vi "openOrigin.vi"   [LabVIEW 2015]
uses:
  <vilib>/registry/registry.llb/Registry RtKey.ctl
  <vilib>/registry/registry.llb/Registry SAM.ctl
  <vilib>/registry/registry.llb/Registry View.ctl
  <vilib>/registry/registry.llb/Read Registry Value Simple STR.vi
types:
  T1 = typedef "Registry View.ctl" = u16
  T2 = typedef "Registry SAM.ctl" = enum32{"KEY_QUERY_VALUE", "KEY_SET_VALUE", "KEY_CREATE_SUB_KEY", "KEY_ENUMERATE_SUB_KEYS", "KEY_NOTIFY", "KEY_CREATE_LINK", "KEY_READ", "KEY_WRITE", "KEY_ALL_ACCESS", "KEY_READ | KEY_WRITE"}
  T3 = typedef "Registry RtKey.ctl" = enum32{"HKEY_CLASSES_ROOT", "HKEY_CURRENT_USER", "HKEY_LOCAL_MACHINE", "HKEY_USERS", "HKEY_PERFORMANCE_DATA", "HKEY_CURRENT_CONFIG", "HKEY_DYN_DATA"}
  T4 = typedef "Registry refnum.ctl" = refnum<k1>
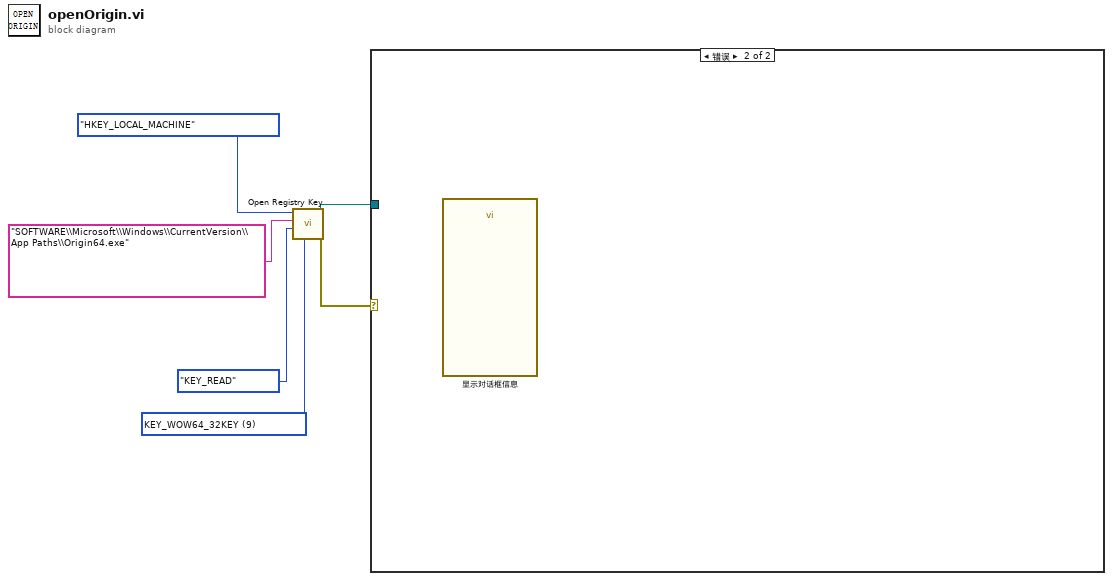
[diagram p0: block diagram]
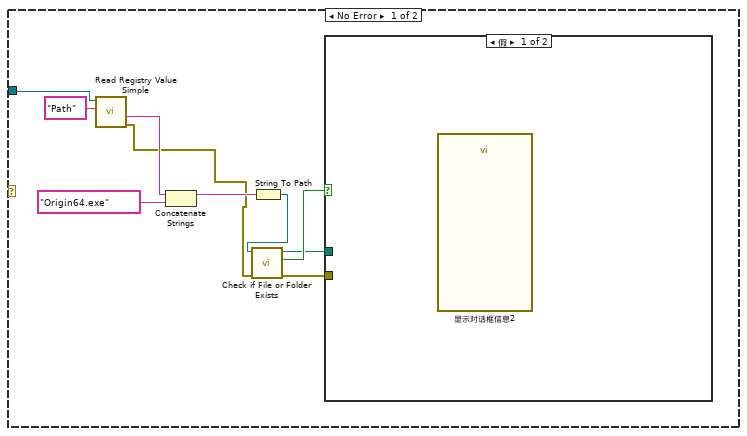
[diagram p2: hidden frame]
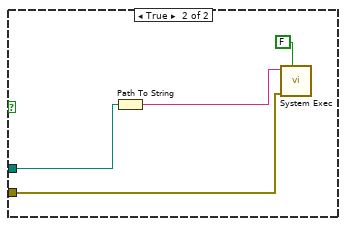
[diagram p3: hidden frame]
diagram:
  w3 = T1 9 items=["Default"=0, "KEY_WOW64_64KEY"=8, "KEY_WOW64_32KEY"=9] ("registry view")
  n1 = call <vilib>:"Open Registry Key.vi"("registry view"=w3, "security access mask (KEY_READ | KEY_WRITE)"=Registry_SAM."KEY_READ", "subkey"="SOFTWARE\\Microsoft\\Windows\\CurrentVersion\\App Paths\\Origin64.exe", "root key (HKEY_LOCAL_MACHINE)"=Registry_RtKey."HKEY_LOCAL_MACHINE") -> ("error out"=w1:errorcluster, "refnum out"=w2:T4)  [unwired: 6 in]
  n2 = case shown="错误" w1 {
    tunnel: w2 -> [w16 _]
    frame No Error {
      n3 = call-poly <vilib>:"Read Registry Value Simple.vi"("value"="Path", "refnum"=w16) -> ("error out"=w8:errorcluster, "String/Binary data"=w14:string)  [unwired: 4 in, 2 out]
      n4 = Concatenate Strings(w14, "Origin64.exe" ("字符串")) -> (w12:string)
      n5 = String To Path(string=w12) -> (path=w11:path)
      n6 = call <vilib>:"Check if File or Folder Exists.vi"("error in (no error)"=w8, "path"=w11) -> ("error out"=w7:errorcluster, "file or folder exists?"=w10:bool, "dup path"=w9:path)  [unwired: 7 in]
      n7 = case shown="假" w10 {
        tunnel: w9 -> [_ w19]
        tunnel: w7 -> [_ w18]
        frame False {
          n8 = call "显示对话框信息2"() -> ()  [unwired: 10 in, 2 out]
        }
        frame True {
          n9 = Path To String(path=w19) -> (string=w17:string)
          n10 = call <vilib>:"System Exec.vi"("wait until completion? (T)"=FALSE, "error in (no error)"=w18, "command line"=w17) -> ()  [unwired: 5 in, 4 out]
        }
      }
    }
    frame Error {
      n11 = call "显示对话框信息"() -> ()  [unwired: 10 in, 2 out]
    }
  }
